vi "Initialize.vi"(8 "error in (no error)":errorcluster, 9 "Reset? (T: Yes)":bool=TRUE, 10 "ID Query? (T: Yes)":bool=TRUE, 11 "VISA resource name":refnum<visa-resource-name>) -> (0 "error out":errorcluster, 3 "VISA resource name out":refnum<visa-resource-name>)   [LabVIEW 2015, in "Agilent ENA Series.lvlib"]
doc: "Establishes communication with the instrument and optionally performs an instrument identification query and/or an instrument reset. It also places the instrument in a default state needed for other instrument driver operations. Therefore, call this VI before calling other instrument driver VIs for this instrument. Generally, you need to call the <B>Initialize VI</B> only once at the beginning of an application."
uses:
  Agilent ENA Series.lvlib
panel:
  # "(c) 2005 - 2010 National Instruments.  ALL RIGHTS RESERVED."
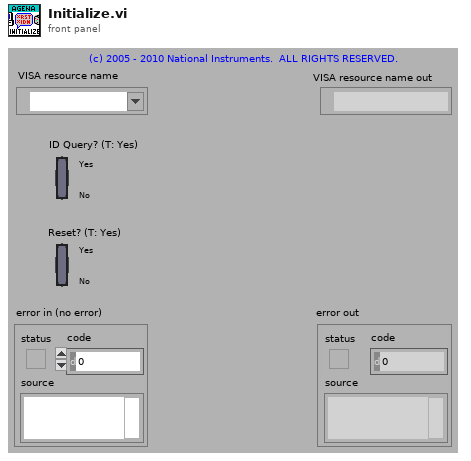
[diagram p1: front panel]
types:
  T1 = cluster{"Status":bool, "Code":i32, "Source (VI Name)":string}
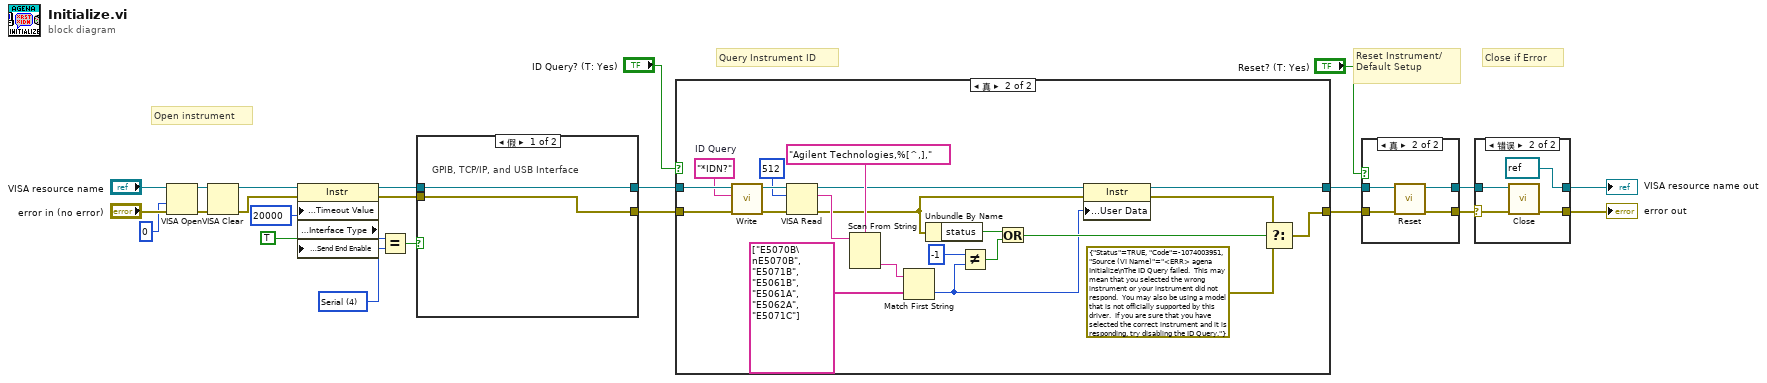
[diagram p0: block diagram]
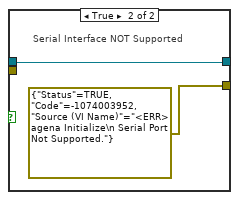
[diagram p2: hidden frame]
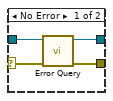
[diagram p3: hidden frame]
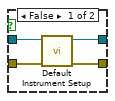
[diagram p4: hidden frame]
diagram:
  w13 = u16 4 items=["GPIB"=1, "VXI"=2, "GPIB-VXI"=3, "Serial"=4, "PXI"=5, "TCPIP"=6, "USB"=7] ("Interface Information:Interface Type")
  # "Close if Error"
  # "Query Instrument ID"
  # "Reset Instrument/\nDefault Setup"
  # "Open instrument"
  n1 = VISA Open(access mode=u32 0, error in (no error)="error in (no error)", VISA resource name="VISA resource name") -> (VISA resource name=w3:refnum<visa-resource-name>, error out=w4:errorcluster)  [unwired: 2 in]
  n2 = VISA Clear(VISA resource name=w3, error in (no error)=w4) -> (VISA resource name out=w2:refnum<visa-resource-name>, error out=w1:errorcluster)
  n3 = property class="Instr"(reference=w2, error in=w1, "General Settings:Timeout Value"=u32 20000, "Message Based Settings:Send End Enable"=TRUE) -> (reference out=w16:refnum<visa-resource-name>, error out=w15:errorcluster, "Interface Information:Interface Type"=w18:u16)
  n4 = Equal?(x=w18, y=w13) -> (x = y?=w14:bool)
  n5 = case shown="假" w14 {
    tunnel: [w26 w28] -> w6
    tunnel: [w25 T1 {"Status"=TRUE, "Code"=-1074003952, "Source (VI Name)"="<ERR> agena Initialize\n Serial Port Not Supported."}] -> w5
    tunnel: w16 -> [w26 w28]
    tunnel: w15 -> [w25 _]
    frame False {
      # "GPIB, TCP/IP, and USB Interface"
    }
    frame True {
      # "Serial Interface NOT Supported"
    }
  }
  n6 = case shown="真" "ID Query? (T: Yes)" {
    tunnel: [w29 w51] -> w23
    tunnel: [w30 w34] -> w24
    tunnel: w6 -> [w30 w49]
    tunnel: w5 -> [w29 w50]
    frame False {
    }
    frame True {
      w41 = "*IDN?"  # ID Query
      n7 = call "Write.vi"("error in (no error)"=w50, "String ()"=w41, "VISA resource name"=w49) -> ("error out"=w46:errorcluster, "VISA resource name out"=w47:refnum<visa-resource-name>)  [unwired: 6 in, 1 out]
      n8 = VISA Read(VISA resource name=w47, byte count=u32 512, error in (no error)=w46) -> (VISA resource name out=w35:refnum<visa-resource-name>, read buffer=w38:string, error out=w33:errorcluster)  [unwired: 1 out]
      n9 = Scan From String(format string="Agilent Technologies,%[^,],", input string=w38) -> (output 1=w37:string)  [unwired: 3 in, 3 out]
      n10 = Match First String(2:string[] ["E5070B\nE5070B", "E5071B", "E5061B", "E5061A", "E5062A", "E5071C"] ("string array"), 3:w37) -> (0:w31:i32)  [unwired: 1 out]
      n11 = Unbundle By Name(w33) -> ("status"=w44:bool)
      n12 = Not Equal?(x=-1, y=w31) -> (x != y?=w48:bool)
      n13 = Or(x=w44, y=w48) -> (x .or. y?=w45:bool)
      n14 = property on="Property Node" class="Instr"(reference=w35, error in=w33, "General Settings:User Data"=w31) -> (reference out=w34:refnum<visa-resource-name>, error out=w32:errorcluster)
      n15 = Select(t=w32, s=w45, f=T1 {"Status"=TRUE, "Code"=-1074003951, "Source (VI Name)"="<ERR> agena Initialize\nThe ID Query failed.  This may mean that you selected the wrong instrument or your instrument did not respond.  You may also be using a model that is not officially supported by this driver.  If you are sure that you have selected the correct instrument and it is responding, try disabling the ID Query."}) -> (s? t:f=w51:T1)
    }
  }
  n16 = case shown="真" "Reset? (T: Yes)" {
    tunnel: w23 -> [w54 w56]
    tunnel: [w53 w59] -> w8
    tunnel: w24 -> [w55 w57]
    tunnel: [w52 w58] -> w9
    frame False {
      n17 = call "Default Instrument Setup.vi"("error in (no error)"=w54, "VISA resource name"=w55) -> ("error out"=w53:errorcluster, "VISA resource name out"=w52:refnum<visa-resource-name>)  [unwired: 8 in]
    }
    frame True {
      n18 = call "Reset.vi"("error in (no error)"=w56, "VISA resource name"=w57) -> ("error out"=w59:errorcluster, "VISA resource name out"=w58:refnum<visa-resource-name>)  [unwired: 8 in]
    }
  }
  n19 = case shown="错误" w8 {
    selector: w8 -> [w61 w65]
    tunnel: w9 -> [w60 w66]
    tunnel: [w63 refnum<visa-resource-name> refnum ("VISA resource name out")] -> w11
    tunnel: [w62 w67] -> w10
    frame No Error {
      n20 = call "Error Query.vi"("error in (no error)"=w61, "VISA resource name"=w60) -> ("error out"=w62:errorcluster, "VISA resource name out"=w63:refnum<visa-resource-name>)  [unwired: 6 in, 2 out]
    }
    frame Error {
      n21 = call "Close.vi"("error in (no error)"=w65, "VISA resource name"=w66) -> ("error out"=w67:errorcluster)  [unwired: 9 in]
    }
  }
  "VISA resource name out" <- w11
  "error out" <- w10
